vi "Get Velocity ESP.vi"(8 "error in (no error)":errorcluster, 9 "Axis (1)":i32=1 min=1 max=3, 10 "VISA resource name":refnum<visa-resource-name>, 11 "ESP302 in":refnum<class "ESP302.lvclass">) -> (0 "error out":errorcluster, 1 "Velocity (units/s)":dbl format="%.4g", 2 "VISA resource name out":refnum<visa-resource-name>, 3 "ESP302 out":refnum<class "ESP302.lvclass">)   [LabVIEW 2020, in "ESP302.lvclass"]
uses:
  ESP302.lvclass
  ESP301.lvclass
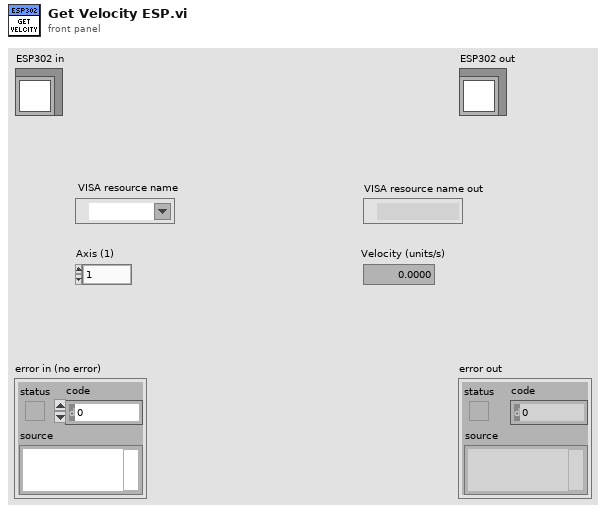
[diagram p1: front panel]
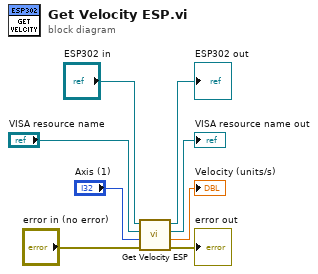
[diagram p0: block diagram]
diagram:
  n1 = call-parent "Get Velocity ESP.vi"("error in (no error)"="error in (no error)", "Axis (1)"="Axis (1)", "VISA resource name"="VISA resource name", "ESP301 in"="ESP302 in") -> ("error out"=→"error out":errorcluster, "Velocity (units/s)"=→"Velocity (units/s)":dbl, "VISA resource name out"=→"VISA resource name out":refnum<visa-resource-name>, "ESP301 out"=→"ESP302 out":refnum<class "ESP302.lvclass">)  [unwired: 4 in]
